vi "MB Mater_Ethernet.vi"() -> ()   [LabVIEW 2014]
uses:
  Program Files/National Instruments/LabVIEW 2014/nimodbus121/86/vi.lib/NI Modbus.llb/MB Modbus Command.ctl
panel:
  in  "Remote Port":u16=502
  in  "Remote IP Address":string="127.0.0.1"
  in  "Stop":bool
  out "Slave Input Registers":u16[](array[numeric]) caption="Slave Input Registers (Read Only)"
  out "Slave Discrete Inputs":bool[](array[boolean])
  in  "Coils to Write":bool[](array[boolean])=[FALSE, FALSE, FALSE, FALSE]
  in  "Registers to Write":u16[](array[numeric])=[0, 0, 0, 0]
  # "MB Ethernet Example Master.vi\n\nInstructions\n1. Run MB Ethernet Example Slave.vi\n2. Run this VI.\n3. Modify the discrete inputs or input registers on the slave -> they're updated on the master.\n4. Modify the coils and registers on the master -> they're updated on the slave."
  # "Data to write to the slave"
  # "Slave Read-only Registers"
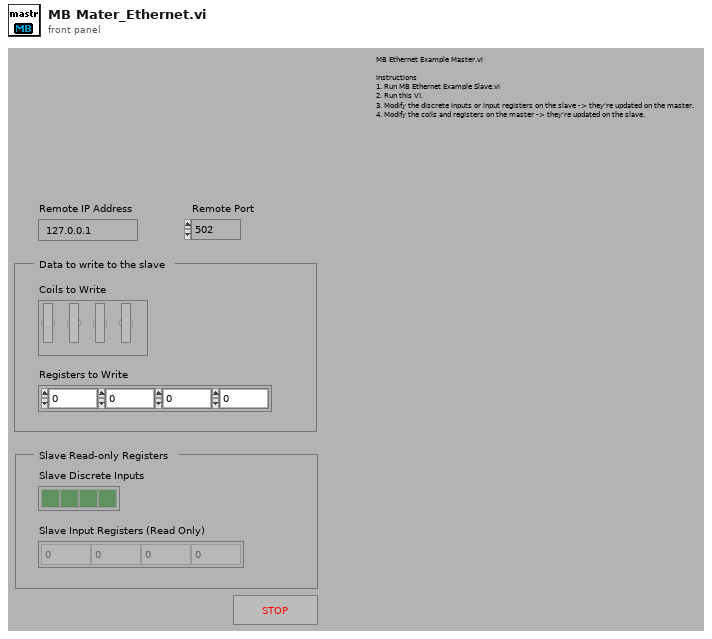
[diagram p1: front panel]
types:
  T1 = typedef "MB Modbus Command.ctl" = cluster{"Function Code":u8, "Starting Address":u16, "Quantity":u16, "Data":u16[], "Discrete":bool[]}
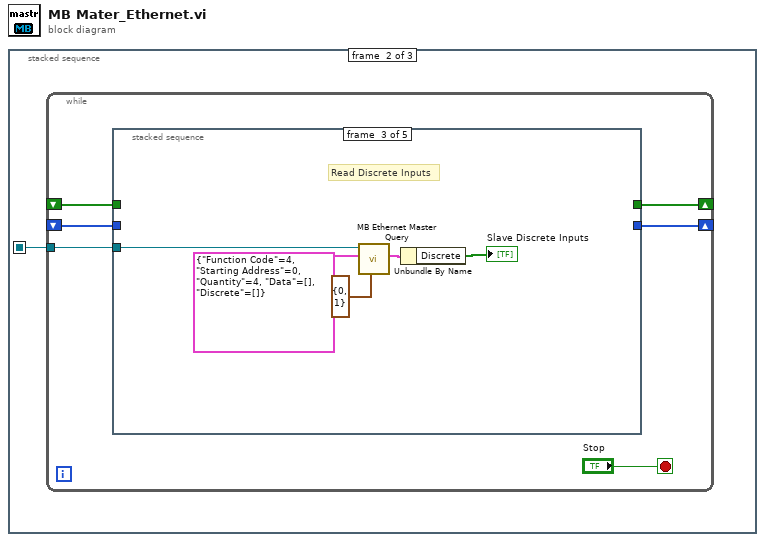
[diagram p0: block diagram]
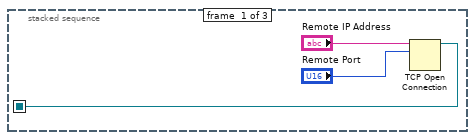
[diagram p2: hidden frame]
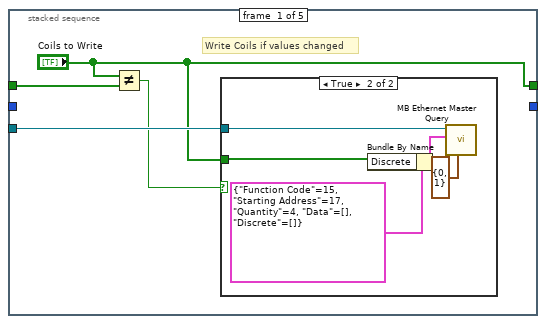
[diagram p3: hidden frame]
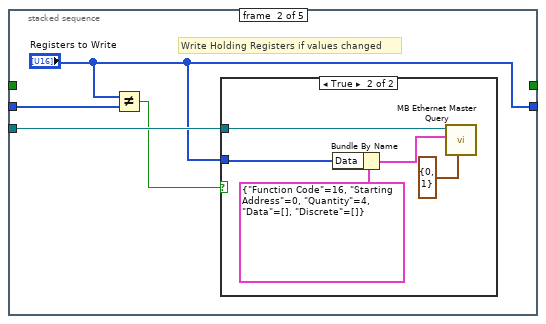
[diagram p5: hidden frame]
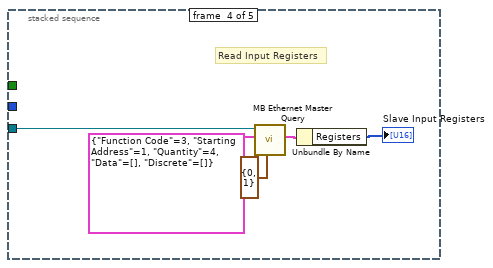
[diagram p7: hidden frame]
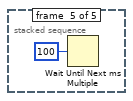
[diagram p8: hidden frame]
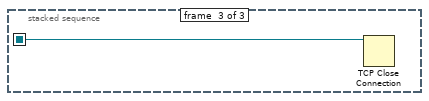
[diagram p9: hidden frame]
diagram:
  n1 = stacked-sequence {
    seq-local: [w1 _ _] -> [_ w4 w40]
    frame #0 {
      n2 = TCP Open Connection(address="Remote IP Address", remote port or service name="Remote Port") -> (connection ID=w1:refnum<k5>)  [unwired: 3 in, 1 out]
    }
    frame #1 {
      n3 = while {
        tunnel: w4 -> [w10]
        shift-right: [w8] -> _
        shift-left: _ -> [w9]
        shift-right: [w6] -> _
        shift-left: _ -> [w7]
        stop <- "Stop" stop-if-true
        n4 = stacked-sequence {
          tunnel: w10 -> [w14 w23 w33 w38 _]
          tunnel: w9 -> [w13 _ _ _ _]
          tunnel: ["Coils to Write" _ _ _ _] -> w8
          tunnel: w7 -> [_ w21 _ _ _]
          tunnel: [_ "Registers to Write" _ _ _] -> w6
          frame #0 {
            # "Write Coils if values changed"
            n5 = Not Equal?(x="Coils to Write", y=w13) -> (x != y?=w11:bool)
            n6 = case shown="True" w11 {
              tunnel: w14 -> [_ w17]
              tunnel: "Coils to Write" -> [_ w16]
              frame False {
              }
              frame True {
                n7 = Bundle By Name(cluster=T1 {"Function Code"=15, "Starting Address"=17, "Quantity"=4, "Data"=[], "Discrete"=[]} ("MODBUS Command"), "Discrete"=w16) -> (w18:T1)
                n8 = call "MB Ethernet Master Query.vi"("MBAP Header"=cluster{"Transaction ID":u16, "Unit ID":u8} {"Transaction ID"=0, "Unit ID"=1}, "Modbus Command"=w18, "TCP Connection Refnum in"=w17) -> ()  [unwired: 4 in, 5 out]
              }
            }
          }
          frame #1 {
            # "Write Holding Registers if values changed"
            n9 = Not Equal?(x="Registers to Write", y=w21) -> (x != y?=w22:bool)
            n10 = case shown="True" w22 {
              tunnel: w23 -> [_ w26]
              tunnel: "Registers to Write" -> [_ w25]
              frame False {
              }
              frame True {
                n11 = Bundle By Name(cluster=T1 {"Function Code"=16, "Starting Address"=0, "Quantity"=4, "Data"=[], "Discrete"=[]} ("MODBUS Command"), "Data"=w25) -> (w27:T1)
                n12 = call "MB Ethernet Master Query.vi"("MBAP Header"=cluster{"Transaction ID":u16, "Unit ID":u8} {"Transaction ID"=0, "Unit ID"=1}, "Modbus Command"=w27, "TCP Connection Refnum in"=w26) -> ()  [unwired: 4 in, 5 out]
              }
            }
          }
          frame #2 {
            # "Read Discrete Inputs"
            n13 = call "MB Ethernet Master Query.vi"("MBAP Header"=cluster{"Transaction ID":u16, "Unit ID":u8} {"Transaction ID"=0, "Unit ID"=1}, "Modbus Command"=T1 {"Function Code"=4, "Starting Address"=0, "Quantity"=4, "Data"=[], "Discrete"=[]} ("MODBUS Command"), "TCP Connection Refnum in"=w33) -> ("Registers"=w32:cluster{"Registers":u16[], "Discrete":bool[]})  [unwired: 4 in, 4 out]
            n14 = Unbundle By Name(w32) -> ("Discrete"=→"Slave Discrete Inputs":bool[])
          }
          frame #3 {
            # "Read Input Registers"
            n15 = call "MB Ethernet Master Query.vi"("MBAP Header"=cluster{"Transaction ID":u16, "Unit ID":u8} {"Transaction ID"=0, "Unit ID"=1}, "Modbus Command"=T1 {"Function Code"=3, "Starting Address"=1, "Quantity"=4, "Data"=[], "Discrete"=[]} ("MODBUS Command"), "TCP Connection Refnum in"=w38) -> ("Registers"=w37:cluster{"Registers":u16[], "Discrete":bool[]})  [unwired: 4 in, 4 out]
            n16 = Unbundle By Name(w37) -> ("Registers"=→"Slave Input Registers":u16[])
          }
          frame #4 {
            n17 = Wait Until Next ms Multiple(millisecond multiple=u32 100) -> ()  [unwired: 1 out]
          }
        }
      }
    }
    frame #2 {
      n18 = TCP Close Connection(connection ID=w40) -> ()  [unwired: 2 in, 2 out]
    }
  }
